vi "Configure Custom Trigger.vi"(0 "device session in":refnum<class "Device Session.lvclass">, 5 "TrigCfg":T1(array[cluster]), 11 "error in":errorcluster) -> (4 "device session out":refnum<class "Device Session.lvclass">, 15 "error out":errorcluster)   [LabVIEW 2021, in "Device Session.lvclass"]
doc: "Configures the edge trigger for the selected channel. You can specify the trigger level, hysteresis, and trigger slope.\n\n<B>Input Parameters</B>\n\n<B>device session in</B> is a reference to the Device Session object, which contains a session to each instrument design library used in this sample project. This parameter is obtained from the 'Open Session' VI.\n\n<B>trigger source</B> specifies the channel to monitor for trigger conditions.\n\n<B>trigger slope</B> specifies whether the oscilloscope should trigger on a rising edge or a falling edge.\n\n<B>trigger level (V)</B> specifies the voltage threshold for the trigger.\n\n<B>hysteresis (%fs)</B> specifies in volts the size of the hysteresis window on either side of the specified 'level'. The oscilloscope triggers when the 'trigger source' signal passes through the 'hysteresis level' you specify with this parameter, has the specified 'trigger slope', and passes through the specified 'level'.\n\n<B>instance</B> specifies either instance A or B of the trigger to use.\n\n<B>error in</B> describes error conditions that occur before this node runs. This input provides standard 'error in' functionality.\n\n<B>Output Parameters</B>\n\n<B>device session out</B> passes a reference to the session to the next VI.\n\n<B>error out</B> contains error information. This output provides standard 'error out' functionality."
uses:
  Device Session.lvclass
  Device Session.lvclass/Device Session.ctl
  <vilib>/rvi/interface/nirviReadWriteControl/nirviReadWriteControl.xnode
  FPGA Refnum.ctl
  NiFpgaLv.dll
  <vilib>/Utility/error.llb/Error Cluster From Error Code.vi
  <vilib>/rvi/interface/Simulation/niFpgaSimulationCallBeginRW.vi
  <vilib>/rvi/errors/niLvFpgaAdjustHostInterfaceError.vi
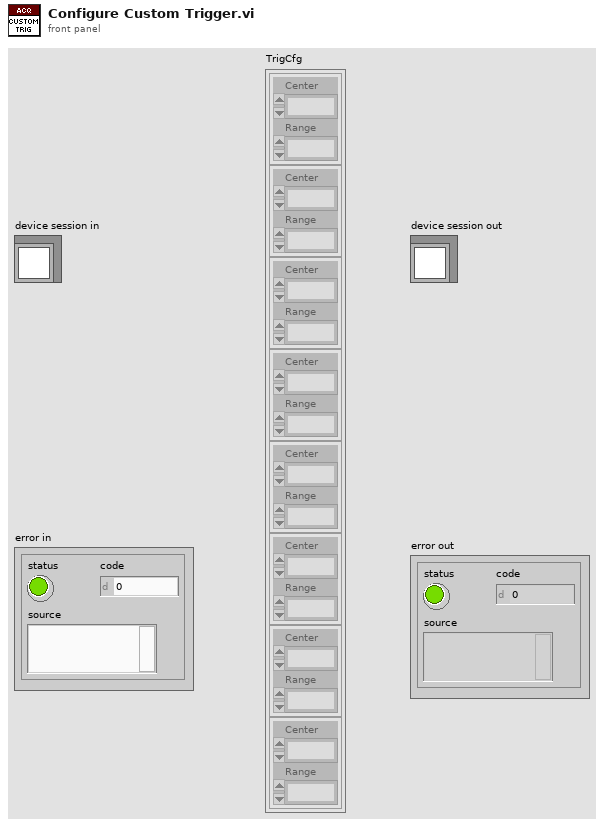
[diagram p1: front panel]
types:
  T1 = cluster{"Center":fxp<+/-,24,1>, "Range":fxp<+,24,1>}[]
  T2 = cluster{"channel":u8, "Center":fxp<+/-,24,1>, "Range":fxp<+,24,1>}
  T3 = typedef "Device Session.lvclass/Device Session Object.ctl" = cluster{"fpga reference":T4, "reg bus":refnum<class "niInstr FIFO Register Bus v1 Host.lvclass">, "subsystem map":refnum<class "niInstr Subsystem Map v1 Host.lvclass">, "cal data":refnum<class "niHSAI Cal Data v1 Host.lvclass">, "config":refnum<class "niHSAI Group A Config v1 Host.lvclass">, "acquisition 0":refnum<class "niInstr Multirecord Acquisition v1 Host.lvclass">, "acquisition 1":refnum<class "niInstr Multirecord Acquisition v1 Host.lvclass">, "number of selected acq channels":u8, "selected acq channels":bool[], "number of channels":u32, "configured channels":bool[], "acq configuration":cluster{"number of samples":u64, "number of records":u64, "pretrigger samples":u64}, "actual channel configuration":T5[], "sample clock rate (Hz)":dbl, "scaling coefficients":T9[]}
  T4 = typedef "Device Session.lvclass/FPGA Refnum.ctl" = refnum<k20>
  T5 = typedef "niHSAI Types v1 Host.lvlib/Channel Configuration.ctl" = cluster{"channel":u32, "coupling":T6, "impedance":T7, "bandwidth":T8, "vertical range":dbl, "vertical offset":dbl}
  T6 = typedef "niHSAI Types v1 Host.lvlib/Coupling.ctl" = enum8{"Default", "DC", "AC"}
  T7 = typedef "niHSAI Types v1 Host.lvlib/Impedance.ctl" = enum8{"Default", "1 mega ohm", "50 ohm"}
  T8 = typedef "niHSAI Types v1 Host.lvlib/Bandwidth.ctl" = enum8{"Default", "Full Bandwidth", "Anti-alias Filter", "150 MHz"}
  T9 = typedef "niInstr Multirecord Acquisition v1 Host.lvclass/Scaling Coefficient.ctl" = cluster{"gain":dbl, "offset":dbl}
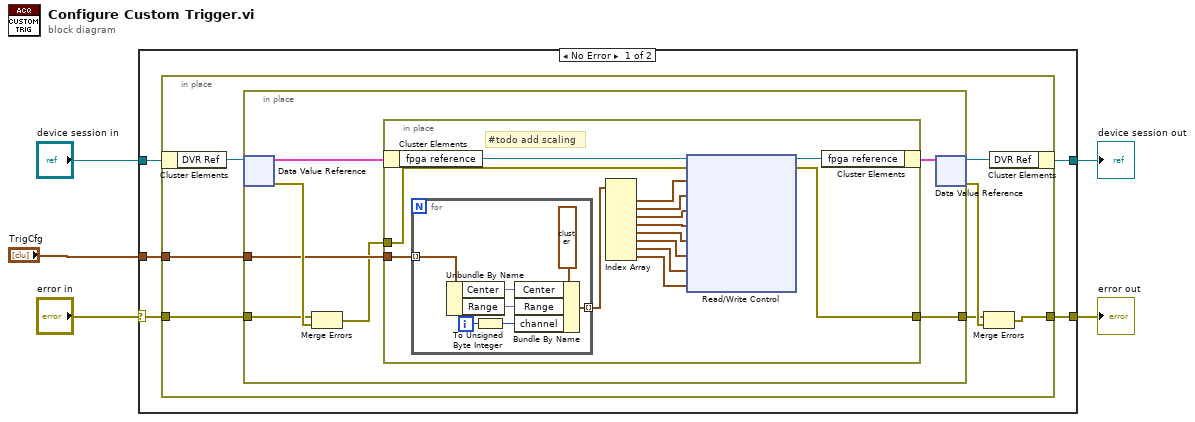
[diagram p0: block diagram]
diagram:
  n1 = case shown="No Error" "error in" {
    selector: "error in" -> [w10 w47]
    tunnel: "device session in" -> [w8 w46]
    tunnel: [w7 w46] -> w4
    tunnel: [w9 w47] -> w5
    tunnel: "TrigCfg" -> [w6 _]
    frame No Error {
      n2 = in-place {
        in-place-border: w10 -> [w17]
        in-place-border: [w14] -> w9
        in-place-border: w6 -> [w11]
        n3 = in-place-cluster #1(w8) -> ("DVR Ref"=w13:refnum<data-value>)
        n4 = in-place {
          in-place-border: w17 -> [w23]
          in-place-border: [w22] -> w15
          in-place-border: w11 -> [w19]
          n5 = in-place-dvr #2(w13) -> (w21:T3, w24:errorcluster)
          n6 = Merge Errors(w23, w24) -> (w18:errorcluster)
          n7 = in-place {
            in-place-border: [w35] -> w22
            in-place-border: w19 -> [w34]
            in-place-border: w18 -> [w37]
            # "#todo add scaling"
            n8 = in-place-cluster #3(w21) -> ("fpga reference"=w38:T4)
            n9 = for {
              tunnel: w34 -> [w42] mode=indexing
              tunnel: [w39] -> w33 mode=indexing
              i -> [w44]
              n10 = Unbundle By Name(w42) -> ("Center"=w41:fxp<+/-,24,1>, "Range"=w40:fxp<+,24,1>)
              n11 = To Unsigned Byte Integer(number=w44) -> (unsigned 8bit integer=w43:u8)
              n12 = Bundle By Name(cluster=T2 {"channel"=0, "Center"=0.0, "Range"=0.0} ("Trigger Settings 0"), "Center"=w41, "Range"=w40, "channel"=w43) -> (w39:T2)
            }
            n13 = Index Array(array=w33) -> (element #1=w32:T2, element #2=w31:T2, element #3=w30:T2, element #4=w29:T2, element #5=w28:T2, element #6=w27:T2, element #7=w26:T2, element #8=w25:T2)  [unwired: 8 in]
            n14 = xnode "Read/Write Control"("FPGA VI Reference In"=w38, "error in"=w37, "Trigger Settings 0"=w32, "Trigger Settings 1"=w31, "Trigger Settings 2"=w30, "Trigger Settings 3"=w29, "Trigger Settings 4"=w28, "Trigger Settings 5"=w27, "Trigger Settings 6"=w26, "Trigger Settings 7"=w25) -> ("FPGA VI Reference Out"=w36:T4, "error out"=w35:errorcluster)
            n15 = in-place-cluster #3("fpga reference"=w36) -> (w20:T3)
          }
          n16 = in-place-dvr #2(w20) -> (w12:refnum<data-value>, w16:errorcluster)
        }
        n17 = Merge Errors(w15, w16) -> (w14:errorcluster)
        n18 = in-place-cluster #1("DVR Ref"=w12) -> (w7:refnum<class "Device Session.lvclass">)
      }
    }
    frame Error {
    }
  }
  "error out" <- w5
  "device session out" <- w4
